vi "GCD_Euclidean_1.vi"(1 "integer 2":i32, 2 "integer 1":i32) -> (0 "gcd":i32)   [LabVIEW 2020]
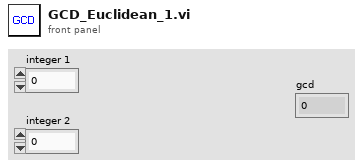
[diagram p1: front panel]
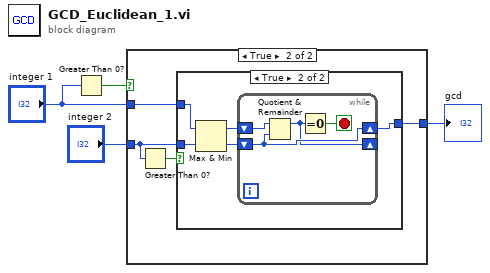
[diagram p0: block diagram]
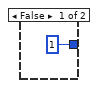
[diagram p2: hidden frame]
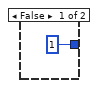
[diagram p3: hidden frame]
diagram:
  n1 = Greater Than 0?(x="integer 1") -> (x > 0?=w4:bool)
  n2 = case shown="True" w4 {
    tunnel: "integer 2" -> [_ w7]
    tunnel: "integer 1" -> [_ w8]
    tunnel: [1 w6] -> w1
    frame False {
    }
    frame True {
      n3 = Greater Than 0?(x=w7) -> (x > 0?=w9:bool)
      n4 = case shown="True" w9 {
        tunnel: w8 -> [_ w15]
        tunnel: w7 -> [_ w14]
        tunnel: [1 w11] -> w6
        frame False {
        }
        frame True {
          n5 = Max & Min(x=w15, y=w14) -> (max(x,y)=w13:i32, min(x,y)=w12:i32)
          n6 = while {
            shift-right: [w16] -> _
            shift-left: w12 -> [w18]
            shift-right: [w18] -> w11
            shift-left: w13 -> [w19]
            stop <- w17 stop-if-true
            n7 = Quotient & Remainder(x=w19, y=w18) -> (x-y*floor(x/y)=w16:i32)  [unwired: 1 out]
            n8 = Equal To 0?(x=w16) -> (x = 0?=w17:bool)
          }
        }
      }
    }
  }
  "gcd" <- w1
